vi "test Import Error when No Channels.vi"(8 "error in":errorcluster, 11 "TestCase in":refnum<class "1553 Parameters Import.lvclass">) -> (0 "error out":errorcluster, 3 "TestCase out":refnum<class "1553 Parameters Import.lvclass">)   [LabVIEW 2020, in "1553 Parameters Import.lvclass"]
uses:
  1553 Parameters Import.lvclass
  <vilib>/Utility/xml.llb/Write to XML File(string).vi
  <vilib>/addons/_JKI Toolkits/VI Tester/TestCase.llb/TestCase.lvclass
  Import/MIL-STD 1553 Import.lvlib
  C:/Program Files (x86)/National Instruments/LabVIEW 2020/vi.lib/addons/_JKI Toolkits/VI Tester/TestCase.llb/TestCase.lvclass
  C:/Git/niveristand-ballard-milStd1553-custom-device/Source/Custom Device Support/Tests/Unit/Import/1553 Parameters Import.lvclass
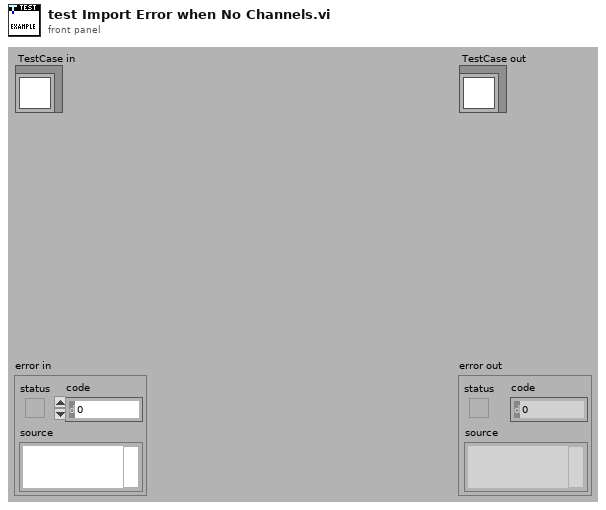
[diagram p1: front panel]
types:
  T1 = typedef "1553 Channel.ctl" = cluster{"HW channel":u16, "terminals":T2[], "messages":T4[], "acyclic frame names":string[]}
  T2 = typedef "Terminal Name and Address.ctl" = cluster{"name":string, "terminal address":T3}
  T3 = typedef "Address.ctl" = u16
  T4 = typedef "Message Definition.ctl" = cluster{"name":string, "message type":T5, "endpoint Rx":T6, "endpoint Tx":T6, "mode code":u16, "number of words":u16, "parameters":cluster{"name":string, "default value":dbl, "unit":string, "parameter definition":T7}[], "create timestamp channel":bool}
  T5 = typedef "Message Type.ctl" = string
  T6 = typedef "Terminal Endpoint.ctl" = cluster{"terminal address":T3, "subaddress":T3}
  T7 = typedef "Parameter Definition.ctl" = cluster{"start index":i32, "size (bits)":i32, "encoding":enum16{"BNR", "BCD", "Discrete"}, "signed":bool, "multiplier":dbl, "offset":dbl}
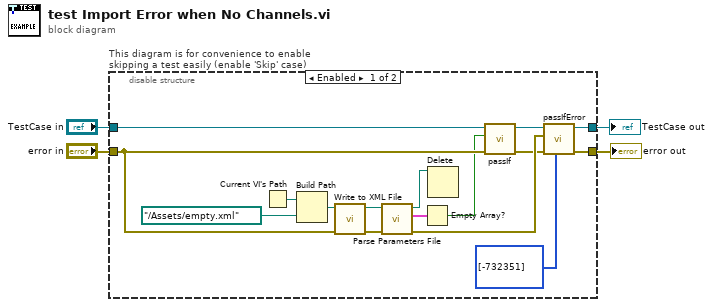
[diagram p0: block diagram]
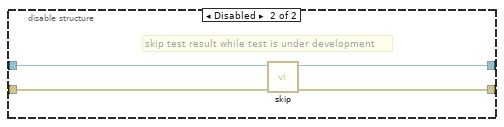
[diagram p2: hidden frame]
diagram:
  n1 = disable-structure "This diagram is for convenience to enable skipping a test easily (enable 'Skip' case)" shown="Enabled" {
    disable-tunnel: "TestCase in" -> [w10 w24]
    disable-tunnel: [w20 w22] -> w1
    disable-tunnel: [w19 w23] -> w3
    disable-tunnel: "error in" -> [w12 w21]
    frame Enabled {
      n2 = Current VI's Path() -> (path=w6:path)
      n3 = Build Path(base path=w6, name or relative path=path "../Assets/empty.xml") -> (appended path=w18:path)
      n4 = call-poly <vilib>:"Write to XML File.vi"("error in (no error)"=w12, "XML File Path"=w18) -> ("error out"=w16:errorcluster, "XML File Path(duplicate)"=w17:path)  [unwired: 7 in, 1 out]
      n5 = call "Parse Parameters File.vi"("error in"=w16, "path to XML document"=w17) -> ("error out"=w15:errorcluster, "1553 channels"=w9:T1[], "path to XML document out"=w7:path)  [unwired: 7 in]
      n6 = Empty Array?(array=w9) -> (empty?=w8:bool)
      n7 = Delete(path (use dialog)=w7) -> ()  [unwired: 4 in, 3 out]
      n8 = call-dynamic "passIf.vi"("error in (no error)"=w12, "pass"=w8, "TestCase in"=w10) -> ("error out"=w13:errorcluster, "TestCase out"=w11:refnum<class "1553 Parameters Import.lvclass">)  [unwired: 7 in]
      n9 = call-dynamic "passIfError.vi"("passing error codes (default = any error code)"=i32[] [-732351], "error in (no error)"=w13, "error"=w15, "TestCase in"=w11) -> ("error out"=w19:errorcluster, "TestCase out"=w20:refnum<class "1553 Parameters Import.lvclass">)  [unwired: 6 in]
    }
    frame Disabled {
      # "skip test result while test is under development"
      n10 = call <vilib>:"skip.vi"("error in (no error)"=w21, "TestCase in"=w24) -> ("error out"=w23:errorcluster, "TestCase out"=w22:refnum<class "1553 Parameters Import.lvclass">)  [unwired: 8 in]
    }
  }
  "error out" <- w3
  "TestCase out" <- w1
